vi "Gamepad Values.vi"() -> (0 "Xbox":T1)   [LabVIEW 2014]
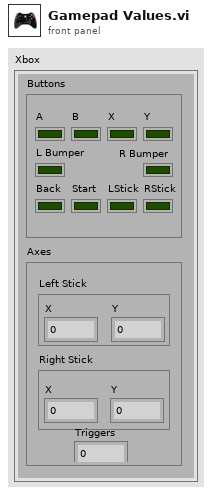
[diagram p1: front panel]
types:
  T1 = cluster{"Buttons":cluster{"A":bool, "B":bool, "X":bool, "Y":bool, "L Bumper":bool, "R Bumper":bool, "Back":bool, "Start":bool, "LStick":bool, "RStick":bool}, "Axes":cluster{"Left Stick":cluster{"X":dbl, "Y":dbl}, "Right Stick":cluster{"X":dbl, "Y":dbl}, "Triggers":dbl}}
  T2 = cluster{"Boolean":bool, "Boolean":bool, "Boolean":bool, "Boolean":bool, "Boolean":bool, "Boolean":bool, "Boolean":bool, "Boolean":bool, "Boolean":bool, "Boolean":bool}
  T3 = cluster{cluster{"Numeric":dbl, "Numeric":dbl}, cluster{"Numeric":dbl, "Numeric":dbl}, "Numeric":dbl}
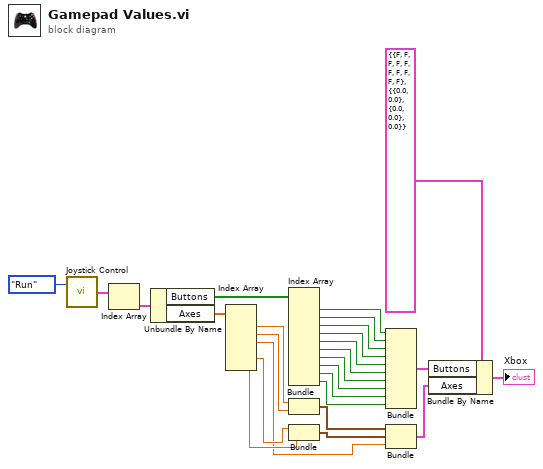
[diagram p0: block diagram]
diagram:
  n1 = call "Joystick Control.vi"("Mode"=enum8{"Start", "Run", "Finish"}."Run") -> ("Joysticks"=w25:cluster{"Buttons":bool[], "Axes":dbl[]}[])  [unwired: 1 in]
  n2 = Index Array(array=w25) -> (element=w24:cluster{"Buttons":bool[], "Axes":dbl[]})  [unwired: 1 in]
  n3 = Unbundle By Name(w24) -> ("Buttons"=w23:bool[], "Axes"=w12:dbl[])
  n4 = Index Array(array=w12) -> (element #1=w11:dbl, element #2=w10:dbl, element #3=w1:dbl, element #5=w3:dbl, element #6=w2:dbl)  [unwired: 6 in, 1 out]
  n5 = Index Array(array=w23) -> (element #1=w22:bool, element #2=w21:bool, element #3=w20:bool, element #4=w18:bool, element #5=w19:bool, element #6=w17:bool, element #7=w16:bool, element #8=w14:bool, element #9=w15:bool, element #10=w13:bool)  [unwired: 10 in]
  n6 = Bundle("Numeric"=w11, "Numeric"=w10) -> (w9:cluster{"Numeric":dbl, "Numeric":dbl})  [unwired: 1 in]
  n7 = Bundle("Numeric"=w3, "Numeric"=w2) -> (w8:cluster{"Numeric":dbl, "Numeric":dbl})  [unwired: 1 in]
  n8 = Bundle("Boolean"=w22, "Boolean"=w21, "Boolean"=w20, "Boolean"=w18, "Boolean"=w19, "Boolean"=w17, "Boolean"=w16, "Boolean"=w14, "Boolean"=w15, "Boolean"=w13) -> (w7:T2)  [unwired: 1 in]
  n9 = Bundle(w9, w8, "Numeric"=w1) -> (w6:T3)  [unwired: 1 in]
  n10 = Bundle By Name(cluster=T1 {"Buttons"={"A"=FALSE, "B"=FALSE, "X"=FALSE, "Y"=FALSE, "L Bumper"=FALSE, "R Bumper"=FALSE, "Back"=FALSE, "Start"=FALSE, "LStick"=FALSE, "RStick"=FALSE}, "Axes"={"Left Stick"={"X"=0.0, "Y"=0.0}, "Right Stick"={"X"=0.0, "Y"=0.0}, "Triggers"=0.0}} ("Xbox"), "Buttons"=w7, "Axes"=w6) -> (→"Xbox":T1)
